vi "Pressure Write.vi"   [LabVIEW 2023, in "Chiller.lvclass"]
uses:
  Chiller.lvclass
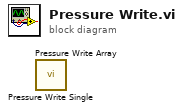
[diagram p0: block diagram]
diagram:
  n1 = call "Pressure Write Single.vi"() -> ()  [unwired: 10 in, 2 out]
  n2 = call "Pressure Write Array.vi"() -> ()  [unwired: 10 in, 2 out]
